vi "Empty_Fruit_Box.vi"() -> (5 "Plug in titles":string[](array[string]), 7 "Plug in values":string[](array[string]))   [LabVIEW 2010]
uses:
  Globals/Meas_global.vi
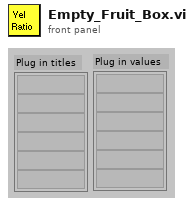
[diagram p1: front panel]
types:
  T1 = typedef "Post_Process.ctl" = enum16{"Take New Data", "Post Process Raw Data File"}
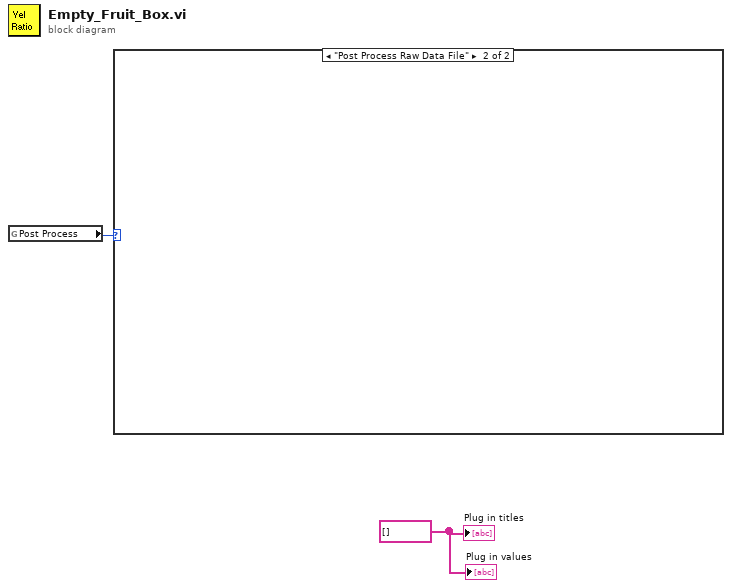
[diagram p0: block diagram]
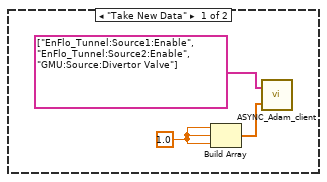
[diagram p2: hidden frame]
diagram:
  w2 = string[] [] ("Plug in titles")
  n1 = global read "Meas_global.vi" "Post Process"() -> (w1:T1)
  n2 = case shown="\"Post Process Raw Data File\"" w1 {
    frame "Take New Data" {
      w3 = 1.0 ("New Value")
      n3 = Build Array(w3, w3, w3) -> (w5:dbl[])
      n4 = call "ASYNC_Adam_client.vi"("Values"=w5, "Channel Names"=string[] ["EnFlo_Tunnel:Source1:Enable", "EnFlo_Tunnel:Source2:Enable", "GMU:Source:Divertor Valve"] ("appended array")) -> ()  [unwired: 2 out]
    }
    frame "Post Process Raw Data File" {
    }
  }
  "Plug in values" <- w2
  "Plug in titles" <- w2
